vi "JSON Unescape.vi"(11 "Escaped String":string) -> (2 "Characters Unescaped?":bool, 3 "String out":string)   [LabVIEW 2019, in "labview_json.lvlib"]
uses:
  labview_json.lvlib
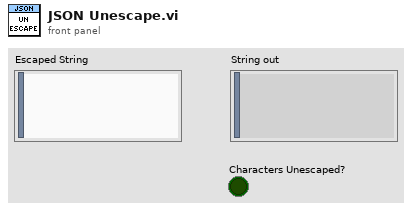
[diagram p1: front panel]
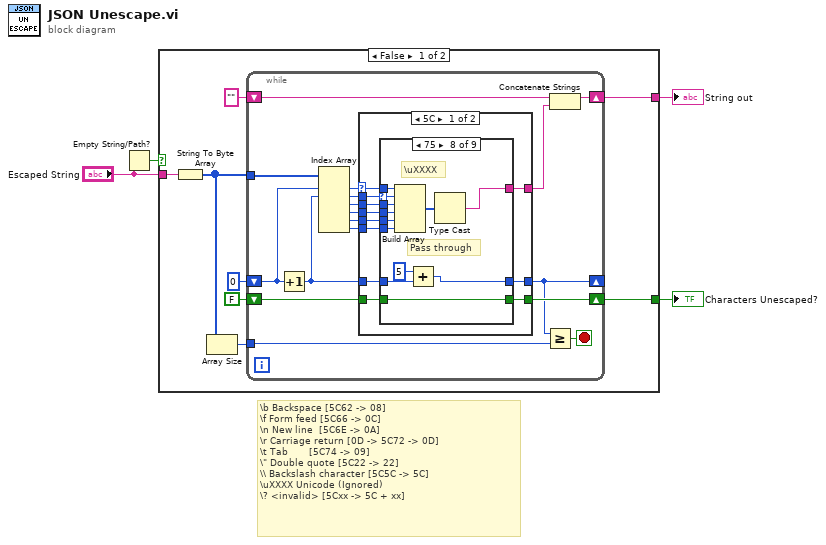
[diagram p0: block diagram]
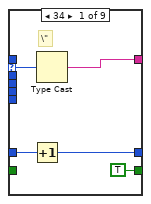
[diagram p2: hidden frame]
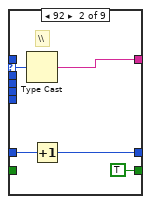
[diagram p3: hidden frame]
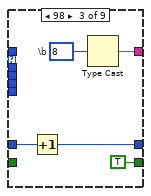
[diagram p4: hidden frame]
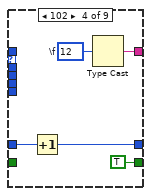
[diagram p5: hidden frame]
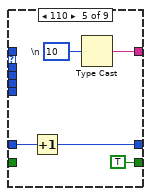
[diagram p6: hidden frame]
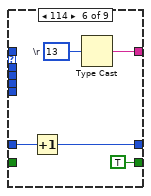
[diagram p7: hidden frame]
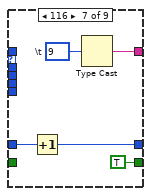
[diagram p8: hidden frame]
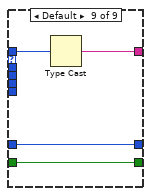
[diagram p9: hidden frame]
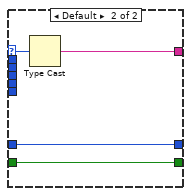
[diagram p10: hidden frame]
diagram:
  # "\\b Backspace [5C62 -> 08]\n\\f Form feed [5C66 -> 0C]\n\\n New line  [5C6E -> 0A]\n\\r Carriage return [0D -> 5C72 -> 0D]\n\\t Tab       [5C74 -> 09]\n\\\" Double quote [5C22 -> 22]\n\\\\ Backslash character [5C5C -> 5C]\n\\uXXXX Unicode (Ignored)\n\\? <invalid> [5Cxx -> 5C + xx]"
  n1 = Empty String/Path?(string/path="Escaped String") -> (empty?=w1:bool)
  n2 = case shown="False" w1 {
    tunnel: "Escaped String" -> [w12 w96]
    tunnel: [w11 _] -> w4
    tunnel: [w5 w96] -> w3
    frame False {
      n3 = String To Byte Array(string=w12) -> (unsigned byte array=w8:u8[])
      n4 = Array Size(array=w8) -> (size(s)=w7:i32)
      n5 = while {
        shift-right: [w28] -> w11
        shift-left: FALSE -> [w27]
        shift-right: [w24] -> _
        shift-left: 0 -> [w25]
        tunnel: w8 -> [w20]
        tunnel: w7 -> [w23]
        shift-right: [w18] -> w5
        shift-left: "" -> [w19]
        stop <- w22 stop-if-true
        n6 = Increment(x=w25) -> (x+1=w21:i32)
        n7 = Index Array(array=w20, index #1=w25, index #2=w21) -> (element #1=w29:u8, element #2=w26:u8, element #3=w16:u8, element #4=w15:u8, element #5=w14:u8, element #6=w13:u8)  [unwired: 4 in]
        n8 = case shown="5C" w29 {
          selector: w29 -> [w39 w93]
          tunnel: [w36 w95] -> w28
          tunnel: w27 -> [w35 w95]
          tunnel: w26 -> [w40 _]
          tunnel: [w38 w94] -> w24
          tunnel: w21 -> [w37 w94]
          tunnel: [w34 w92] -> w17
          tunnel: w16 -> [w33 _]
          tunnel: w15 -> [w32 _]
          tunnel: w14 -> [w31 _]
          tunnel: w13 -> [w30 _]
          frame 92 {
            n9 = case shown="75" w40 {
              selector: w40 -> [w42 w47 _ _ _ _ _ w79 _]
              tunnel: w39 -> [_ _ _ _ _ _ _ w80 w89]
              tunnel: [w43 w48 w53 w58 w63 w68 w73 w85 w91] -> w38
              tunnel: w37 -> [w45 w50 w55 w60 w65 w70 w75 w87 w91]
              tunnel: [TRUE TRUE TRUE TRUE TRUE TRUE TRUE w76 w90] -> w36
              tunnel: w35 -> [_ _ _ _ _ _ _ w76 w90]
              tunnel: [w41 w46 w51 w56 w61 w66 w71 w77 w88] -> w34
              tunnel: w33 -> [_ _ _ _ _ _ _ w84 _]
              tunnel: w32 -> [_ _ _ _ _ _ _ w81 _]
              tunnel: w31 -> [_ _ _ _ _ _ _ w82 _]
              tunnel: w30 -> [_ _ _ _ _ _ _ w83 _]
              frame 34 {
                # "\\\""
                n10 = Increment(x=w45) -> (x+1=w43:i32)
                n11 = Type Cast(x=w42) -> (*(type *) &x=w41:string)  [unwired: 1 in]
              }
              frame 92 {
                # "\\\\"
                n12 = Type Cast(x=w47) -> (*(type *) &x=w46:string)  [unwired: 1 in]
                n13 = Increment(x=w50) -> (x+1=w48:i32)
              }
              frame 98 {
                w52 = u8 8  # \b
                n14 = Increment(x=w55) -> (x+1=w53:i32)
                n15 = Type Cast(x=w52) -> (*(type *) &x=w51:string)  [unwired: 1 in]
              }
              frame 102 {
                w57 = u8 12  # \f
                n16 = Increment(x=w60) -> (x+1=w58:i32)
                n17 = Type Cast(x=w57) -> (*(type *) &x=w56:string)  [unwired: 1 in]
              }
              frame 110 {
                w62 = u8 10  # \n
                n18 = Increment(x=w65) -> (x+1=w63:i32)
                n19 = Type Cast(x=w62) -> (*(type *) &x=w61:string)  [unwired: 1 in]
              }
              frame 114 {
                w67 = u8 13  # \r
                n20 = Increment(x=w70) -> (x+1=w68:i32)
                n21 = Type Cast(x=w67) -> (*(type *) &x=w66:string)  [unwired: 1 in]
              }
              frame 116 {
                w72 = u8 9  # \t
                n22 = Increment(x=w75) -> (x+1=w73:i32)
                n23 = Type Cast(x=w72) -> (*(type *) &x=w71:string)  [unwired: 1 in]
              }
              frame 117 {
                # "Pass through"
                # "\\uXXXX"
                n24 = Build Array(w80, w79, w84, w81, w82, w83) -> (w78:u8[])
                n25 = Add(x=5, y=w87) -> (x+y=w85:i32)
                n26 = Type Cast(x=w78) -> (*(type *) &x=w77:string)  [unwired: 1 in]
              }
              frame Default {
                n27 = Type Cast(x=w89) -> (*(type *) &x=w88:string)  [unwired: 1 in]
              }
            }
          }
          frame Default {
            n28 = Type Cast(x=w93) -> (*(type *) &x=w92:string)  [unwired: 1 in]
          }
        }
        n29 = Greater Or Equal?(x=w24, y=w23) -> (x >= y?=w22:bool)
        n30 = Concatenate Strings(w19, w17) -> (w18:string)
      }
    }
    frame True {
    }
  }
  "String out" <- w3
  "Characters Unescaped?" <- w4
